vi "Clear.vi"(9 "limit":T1, 10 "XYGraphGN":refnum<vi>, 11 "TblRefFormMainShow":refnum<vi>) -> ()   [LabVIEW 2019]
panel:
  out "XY_out":cluster{dbl[], dbl[]}[](graph)
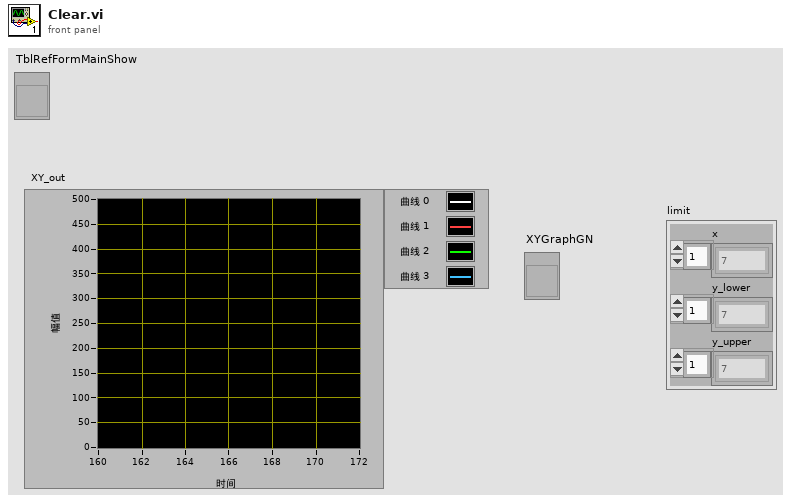
[diagram p1: front panel]
types:
  T1 = cluster{"x":dbl[], "y_lower":dbl[], "y_upper":dbl[]}
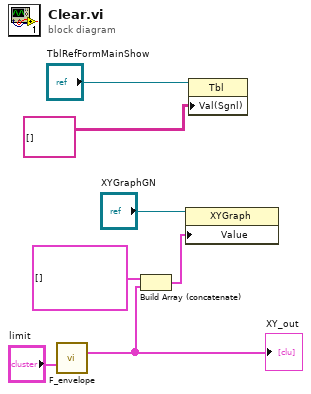
[diagram p0: block diagram]
diagram:
  n1 = call "F_envelope.vi"("limit"="limit") -> ("XY_out"=w3:cluster{dbl[], dbl[]}[])  [unwired: 11 in, 3 out]
  "XY_out" <- w3
  n2 = Build Array (concatenate)(cluster{dbl[], dbl[]}[] [] ("元素"), w3) -> (w1:cluster{dbl[], dbl[]}[])
  n3 = property class="XYGraph"(reference="XYGraphGN", "Value"=w1) -> ()  [unwired: 1 in, 2 out]
  n4 = property class="Tbl"(reference="TblRefFormMainShow", "Val(Sgnl)"=string[][] [] ("值(信号)")) -> ()  [unwired: 1 in, 2 out]
